vi "Configure Modulation Waveform Advanced (Swept-Sine).vi"(0 "VISA resource name":refnum<visa-resource-name>, 1 "Enable Couplings (T: Enable)":bool=TRUE, 2 "Waveform Type (0: Sine)":i32(ring) items=["Sine", "Triangle", "Square", "Ramp"], 3 "Sweep Shape (0: Sawtooth)":i32(ring) items=["Sawtooth", "Triangle"], 5 "Modulation Type (0: Amplitude Modulation)":i32(ring) items=["Amplitude Modulation", "Frequency Modulation", "Phase Modulation", "Low Frequency Output"], 7 "Modulation Path (1: 1)":i32(ring)=1 items=["1"=1, "2"=2], 9 "Start Frequency (400 Hz)":dbl=400.0, 11 "error in (no error)":errorcluster, 12 "Stop Frequency (400 Hz)":dbl=400.0, 13 "Ramp Direction (0: Positive)":i32(ring) items=["Positive", "Negative"]) -> (4 "VISA resource name out":refnum<visa-resource-name>, 15 "error out":errorcluster)   [LabVIEW 2014, in "Agilent PSG MXG Series.lvlib"]
doc: "Configures internal sweep function generator.\n\n<B>Notes:</B>\n1) This VI is valid only in N5171B, N5172B, N5181B, N5182B that install <B>Option UNT</B> and <B>Option 303</B> (AM, FM, phase modulation, and LF output)."
uses:
  Agilent PSG MXG Series.lvlib
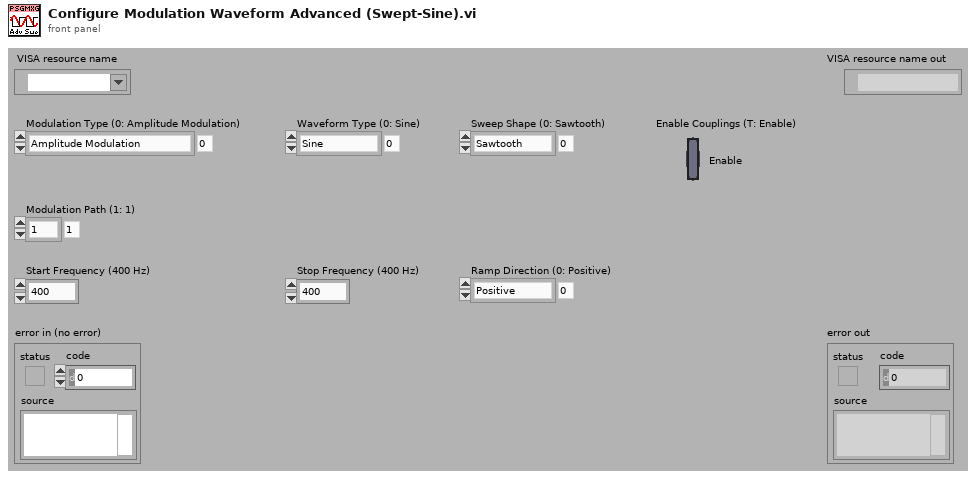
[diagram p1: front panel]
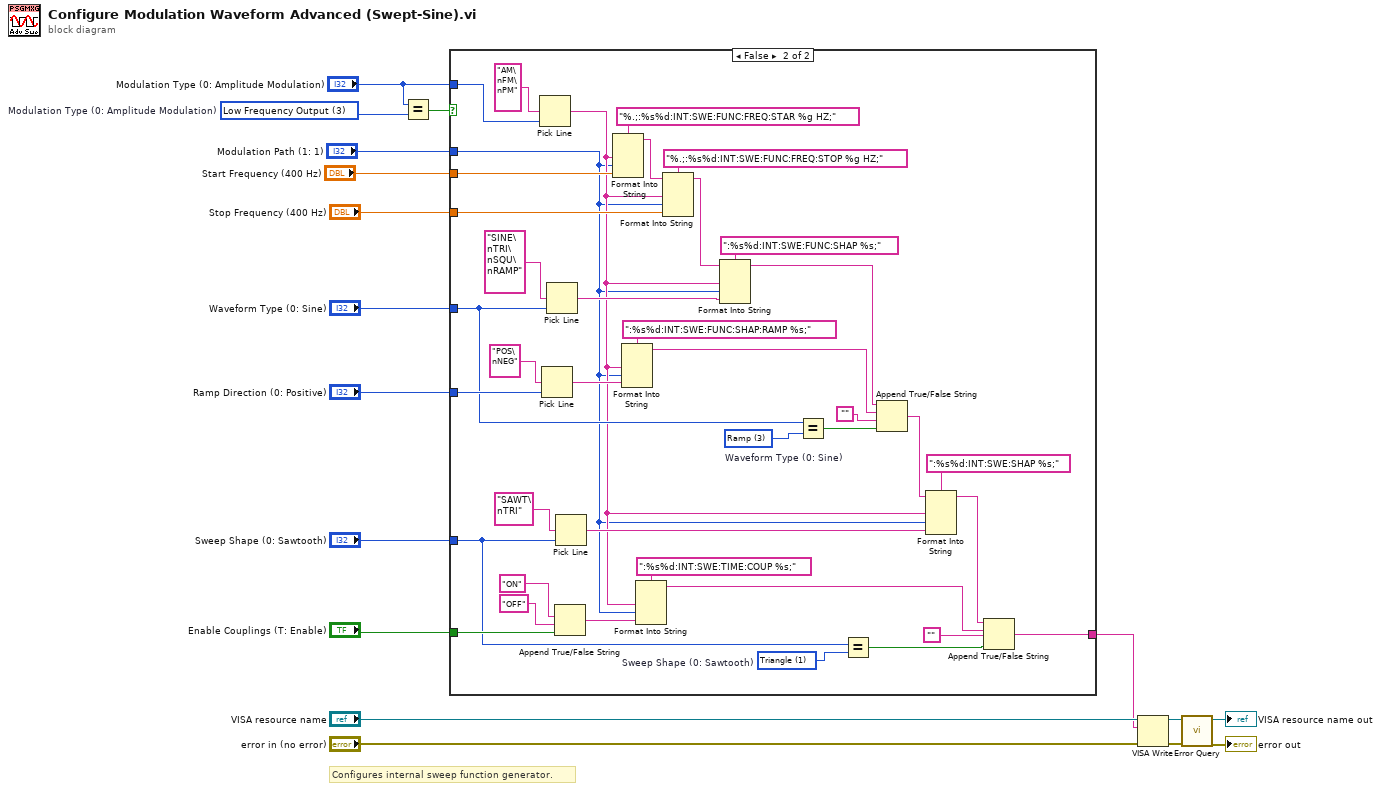
[diagram p0: block diagram]
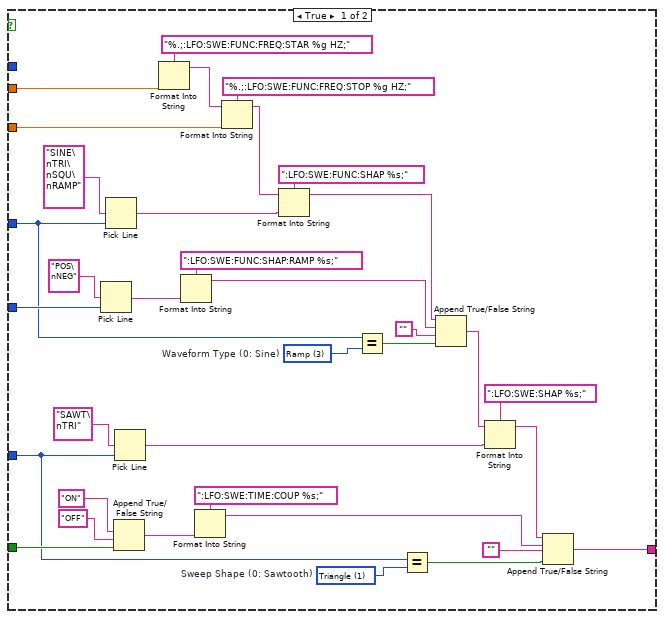
[diagram p2: hidden frame]
diagram:
  w5 = 3 items=["Amplitude Modulation", "Frequency Modulation", "Phase Modulation", "Low Frequency Output"]  # Modulation Type (0: Amplitude Modulation)
  # "Configures internal sweep function generator."
  n1 = Equal?(x="Modulation Type (0: Amplitude Modulation)", y=w5) -> (x = y?=w6:bool)
  n2 = case shown="False" w6 {
    tunnel: "Stop Frequency (400 Hz)" -> [w22 w55]
    tunnel: "Waveform Type (0: Sine)" -> [w35 w69]
    tunnel: "Ramp Direction (0: Positive)" -> [w45 w84]
    tunnel: "Sweep Shape (0: Sawtooth)" -> [w25 w57]
    tunnel: "Enable Couplings (T: Enable)" -> [w39 w78]
    tunnel: "Modulation Type (0: Amplitude Modulation)" -> [_ w75]
    tunnel: "Modulation Path (1: 1)" -> [_ w53]
    tunnel: "Start Frequency (400 Hz)" -> [w23 w74]
    tunnel: [w24 w56] -> w1
    frame True {
      w27 = 1 items=["Sawtooth", "Triangle"]  # Sweep Shape (0: Sawtooth)
      w36 = 3 items=["Sine", "Triangle", "Square", "Ramp"]  # Waveform Type (0: Sine)
      n3 = Pick Line(multi-line string="POS\nNEG", line index=w45) -> (output string=w20:string)  [unwired: 1 out]
      n4 = Pick Line(multi-line string="SINE\nTRI\nSQU\nRAMP", line index=w35) -> (output string=w21:string)  [unwired: 1 out]
      n5 = Append True/False String(1:w39, 2:"OFF", 3:"ON") -> (0:w18:string)  [unwired: 1 out]
      n6 = Pick Line(multi-line string="SAWT\nTRI", line index=w25) -> (output string=w19:string)  [unwired: 1 out]
      n7 = Format Into String(format string="%.;:LFO:SWE:FUNC:FREQ:STAR %g HZ;", w23) -> (resulting string=w51:string)  [unwired: 2 in, 1 out]
      n8 = Format Into String(format string=":LFO:SWE:FUNC:SHAP:RAMP %s;", w20) -> (resulting string=w33:string)  [unwired: 2 in, 1 out]
      n9 = Format Into String(format string=":LFO:SWE:TIME:COUP %s;", w18) -> (resulting string=w28:string)  [unwired: 2 in, 1 out]
      n10 = Format Into String(format string="%.;:LFO:SWE:FUNC:FREQ:STOP %g HZ;", initial string=w51, w22) -> (resulting string=w48:string)  [unwired: 1 in, 1 out]
      n11 = Format Into String(format string=":LFO:SWE:FUNC:SHAP %s;", initial string=w48, w21) -> (resulting string=w32:string)  [unwired: 1 in, 1 out]
      n12 = Equal?(x=w35, y=w36) -> (x = y?=w37:bool)
      n13 = Equal?(x=w25, y=w27) -> (x = y?=w26:bool)
      n14 = Append True/False String(1:w37, 2:"", 3:w33, 4:w32) -> (0:w31:string)
      n15 = Format Into String(format string=":LFO:SWE:SHAP %s;", initial string=w31, w19) -> (resulting string=w30:string)  [unwired: 1 in, 1 out]
      n16 = Append True/False String(1:w26, 2:"", 3:w28, 4:w30) -> (0:w24:string)
    }
    frame False {
      w59 = 1 items=["Sawtooth", "Triangle"]  # Sweep Shape (0: Sawtooth)
      w70 = 3 items=["Sine", "Triangle", "Square", "Ramp"]  # Waveform Type (0: Sine)
      n17 = Pick Line(multi-line string="AM\nFM\nPM", line index=w75) -> (output string=w54:string)  [unwired: 1 out]
      n18 = Pick Line(multi-line string="POS\nNEG", line index=w84) -> (output string=w72:string)  [unwired: 1 out]
      n19 = Pick Line(multi-line string="SINE\nTRI\nSQU\nRAMP", line index=w69) -> (output string=w73:string)  [unwired: 1 out]
      n20 = Append True/False String(1:w78, 2:"OFF", 3:"ON") -> (0:w63:string)  [unwired: 1 out]
      n21 = Pick Line(multi-line string="SAWT\nTRI", line index=w57) -> (output string=w64:string)  [unwired: 1 out]
      n22 = Format Into String(format string="%.;:%s%d:INT:SWE:FUNC:FREQ:STAR %g HZ;", w54, w53, w74) -> (resulting string=w90:string)  [unwired: 2 in, 1 out]
      n23 = Format Into String(format string=":%s%d:INT:SWE:FUNC:SHAP:RAMP %s;", w54, w53, w72) -> (resulting string=w67:string)  [unwired: 2 in, 1 out]
      n24 = Format Into String(format string=":%s%d:INT:SWE:TIME:COUP %s;", w54, w53, w63) -> (resulting string=w60:string)  [unwired: 2 in, 1 out]
      n25 = Format Into String(format string="%.;:%s%d:INT:SWE:FUNC:FREQ:STOP %g HZ;", initial string=w90, w54, w53, w55) -> (resulting string=w87:string)  [unwired: 1 in, 1 out]
      n26 = Format Into String(format string=":%s%d:INT:SWE:FUNC:SHAP %s;", initial string=w87, w54, w53, w73) -> (resulting string=w66:string)  [unwired: 1 in, 1 out]
      n27 = Equal?(x=w69, y=w70) -> (x = y?=w71:bool)
      n28 = Equal?(x=w57, y=w59) -> (x = y?=w58:bool)
      n29 = Append True/False String(1:w71, 2:"", 3:w67, 4:w66) -> (0:w65:string)
      n30 = Format Into String(format string=":%s%d:INT:SWE:SHAP %s;", initial string=w65, w54, w53, w64) -> (resulting string=w62:string)  [unwired: 1 in, 1 out]
      n31 = Append True/False String(1:w58, 2:"", 3:w60, 4:w62) -> (0:w56:string)
    }
  }
  n32 = VISA Write(VISA resource name="VISA resource name", write buffer=w1, error in (no error)="error in (no error)") -> (VISA resource name out=w10:refnum<visa-resource-name>, error out=w9:errorcluster)  [unwired: 1 out]
  n33 = call "Error Query.vi"("error in (no error)"=w9, "VISA resource name"=w10) -> ("error out"=→"error out":errorcluster, "VISA resource name out"=→"VISA resource name out":refnum<visa-resource-name>)  [unwired: 8 out]
